vi "Read.vi"(8 "error in (no error)":errorcluster, 11 "Agilent DMM in":refnum<class "Agilent DMM.lvclass">) -> (0 "error out":errorcluster, 3 "Agilent DMM out":refnum<class "Agilent DMM.lvclass">)   [LabVIEW 2020, in "Agilent DMM.lvclass"]
uses:
  Agilent DMM.lvclass
  D:/Users/Marco Yang/Downloads/LVOOP 2012/LVOOP 2012/DMM/DMM.lvclass
  Agilent DMM.lvclass/Agilent DMM.ctl
  DMM/DMM.lvclass/DMM.ctl
  DMM/DMM.lvclass
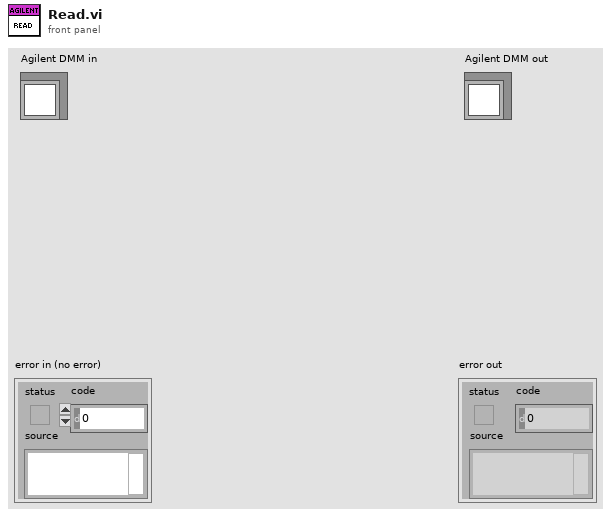
[diagram p1: front panel]
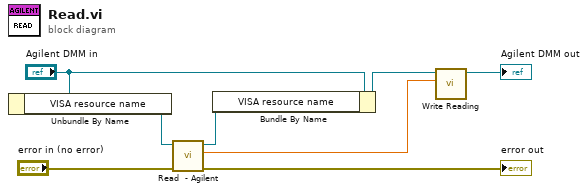
[diagram p0: block diagram]
diagram:
  n1 = Unbundle By Name("Agilent DMM in") -> ("VISA resource name"=w6:refnum<visa-resource-name>)
  n2 = call "Read  - Agilent.vi"("error in (no error)"="error in (no error)", "VISA resource name"=w6) -> ("error out"=→"error out":errorcluster, "Measurement"=w1:dbl, "VISA resource name out"=w5:refnum<visa-resource-name>)  [unwired: 7 in]
  n3 = Bundle By Name(cluster="Agilent DMM in", "VISA resource name"=w5) -> (w3:refnum<class "Agilent DMM.lvclass">)
  n4 = call "Write Reading.vi"("Reading"=w1, "DMM in"=w3) -> ("DMM out"=→"Agilent DMM out":refnum<class "Agilent DMM.lvclass">)  [unwired: 8 in, 1 out]
